vi "Example.vi"() -> ()   [LabVIEW 2019, in "LabErrorUX.lvclass"]
uses:
  LabErrorUX.lvclass
  LabErrorUX.lvclass/LabErrorUX.ctl
  Typedefs/ErrorUX.ctl
panel:
  in  "error in":errorcluster={"status"=TRUE, "code"=7, "source"=""}
  out "ErrorUX":T1
  in  "ErrorUX CSV File Path":path=path "D:/Github/KarthikAbiram/LabErrorUX/Source/SampleLabErrorUX.csv"
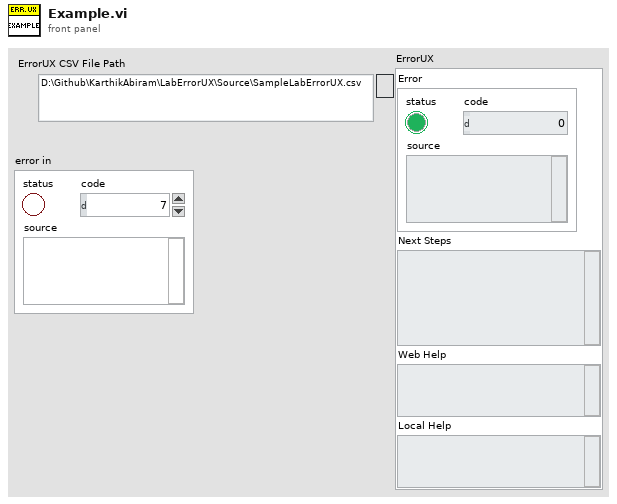
[diagram p1: front panel]
types:
  T1 = typedef "LabErrorUX.lvclass/ErrorUX.ctl" = cluster{"Error":errorcluster, "Next Steps":string, "Web Help":string, "Local Help":string}
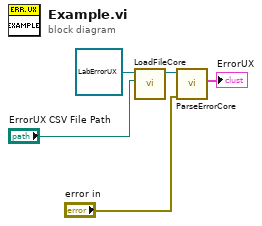
[diagram p0: block diagram]
diagram:
  n1 = call-dynamic "LoadFileCore.vi"("ErrorUX CSV File Path"="ErrorUX CSV File Path", "LabErrorUX in"=refnum<class "LabErrorUX.lvclass"> refnum) -> ("LabErrorUX out"=w4:refnum<class "LabErrorUX.lvclass">)  [unwired: 8 in, 1 out]
  n2 = call-dynamic "ParseErrorCore.vi"("error in (no error)"="error in", "LabErrorUX in"=w4) -> ("ErrorUX"=→"ErrorUX":T1)  [unwired: 7 in, 2 out]
